vi "Write Channel Number.vi"(10 "Channel Number":u8=1, 11 "Power Meter in":refnum<class "Power Meter.lvclass">) -> (3 "Power Meter out":refnum<class "Power Meter.lvclass">)   [LabVIEW 2020, in "Power Meter.lvclass"]
uses:
  Power Meter.lvclass
  Power Meter.lvclass/Power Meter.ctl
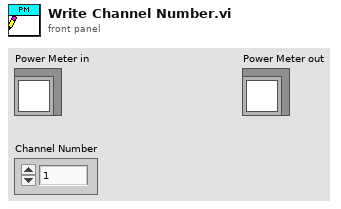
[diagram p1: front panel]
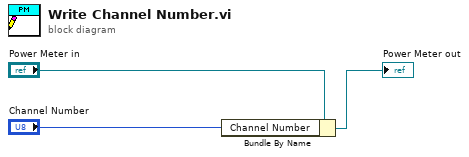
[diagram p0: block diagram]
diagram:
  n1 = Bundle By Name(cluster="Power Meter in", "Channel Number"="Channel Number") -> (→"Power Meter out":refnum<class "Power Meter.lvclass">)
